vi "ID Chain.vi"(11 "Selection":T1) -> (3 "Array":string[](array[string]))   [LabVIEW 2015, in "Read-Write-Signals.xnode"]
uses:
  Read-Write-Signals.xnode
  Read-Write-Signals Selection.ctl
  Read-Write-Signals Item.ctl
  Read-Write-Signals Sub Item.ctl
  Read-Write-Signals Sub Item Type.ctl
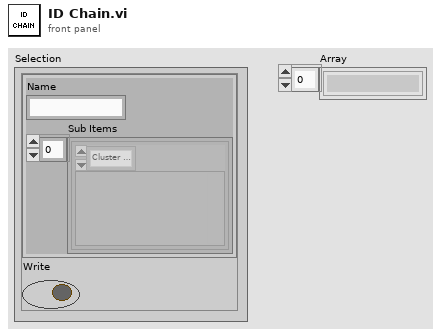
[diagram p1: front panel]
types:
  T1 = typedef "Read-Write-Signals Selection.ctl" = cluster{"Item":T2, "Write":bool}
  T2 = typedef "Read-Write-Signals Item.ctl" = cluster{"Name":string, "Sub Items":T3[]}
  T3 = typedef "Read-Write-Signals Sub Item.ctl" = cluster{"Type":T4, "Value":variant}
  T4 = typedef "Read-Write-Signals Sub Item Type.ctl" = enum8{"Cluster Element", "Array Element", "Subarray"}
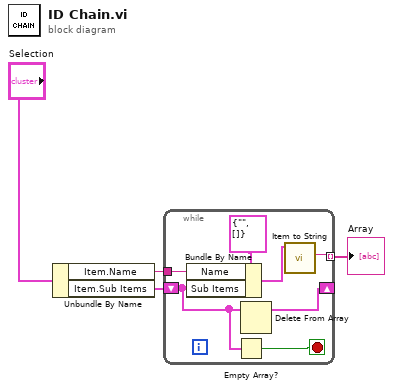
[diagram p0: block diagram]
diagram:
  n1 = Unbundle By Name("Selection") -> ("Item.Name"=w1:string, "Item.Sub Items"=w2:T3[])
  n2 = while {
    tunnel: w1 -> [w11]
    shift-right: [w7] -> _
    shift-left: w2 -> [w6]
    tunnel: [w8] -> w3 mode=indexing
    stop <- w5 stop-if-true
    n3 = Bundle By Name(cluster=T2 {"Name"="", "Sub Items"=[]} ("Item"), "Name"=w11, "Sub Items"=w6) -> (w9:T2)
    n4 = Empty Array?(array=w6) -> (empty?=w5:bool)
    n5 = Delete From Array(array=w6) -> (array with subset deleted=w7:T3[])  [unwired: 2 in, 1 out]
    n6 = call "Item to String.vi"("Item in"=w9) -> ("0 String"=w8:string)  [unwired: 9 in, 1 out]
  }
  "Array" <- w3
